vi "Set Monitoring Session.vi"(8 "error in":errorcluster, 9 "Redundant?":bool, 10 "session_rx_monitor":T1[](array[typedef]) {"Strobe" items=["FDX_MON_STROBE_DIS", "FDX_MON_STROBE_STOP", "FDX_MON_STROBE_START"]; "CaptureMode" items=["FDX_MON_SINGLE ", "FDX_MON_CONTINUOUS", "FDX_MON_SELECTIVE", "FDX_MON_RECORDING", "FDX_MON_REROS", "FDX_MON_HMU"]; "DefaultCronoMode" items=["FDX_RX_DEFAULT_ENA_CNT", "FDX_RX_DEFAULT_MON_ENA_ALL", "FDX_RX_DEFAULT_MON_ENA_GOOD"]}, 11 "Port Section Ref in":T2 format="%.0x") -> (0 "error out":errorcluster, 3 "Item Ref out":T2 format="%.0x")   [LabVIEW 2020, in "AIM ARINC 664 Scripting.lvlib"]
uses:
  AIM ARINC 664 Scripting.lvlib
  <vilib>/NI VeriStand/Custom Device API/Custom Device Item Ref.ctl
  <vilib>/NI VeriStand/Custom Device API/Custom Device API.lvlib
  Shared/session_rx_monitor.ctl
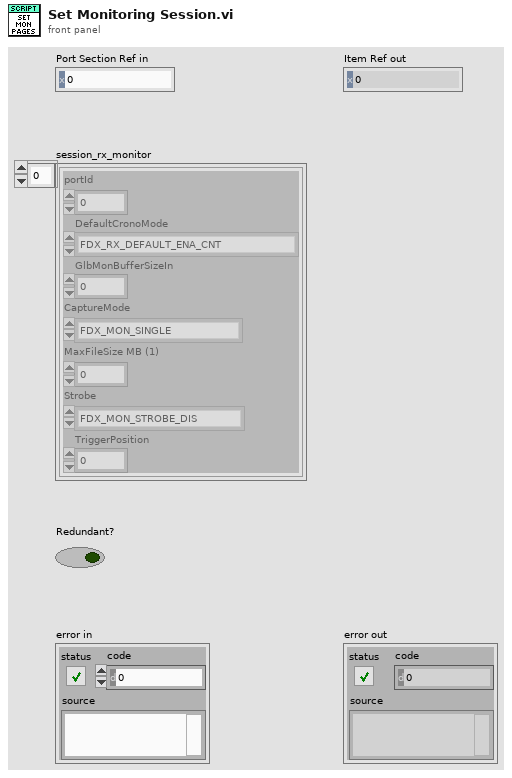
[diagram p1: front panel]
types:
  T1 = typedef "session_rx_monitor.ctl" = cluster{"portId":u32, "DefaultCronoMode":u32, "GlbMonBufferSizeIn":u32, "CaptureMode":u32, "MaxFileSize MB (1)":u32, "Strobe":u32, "TriggerPosition":u32}
  T2 = typedef "Custom Device API.lvlib/Custom Device Item Ref.ctl" = u64
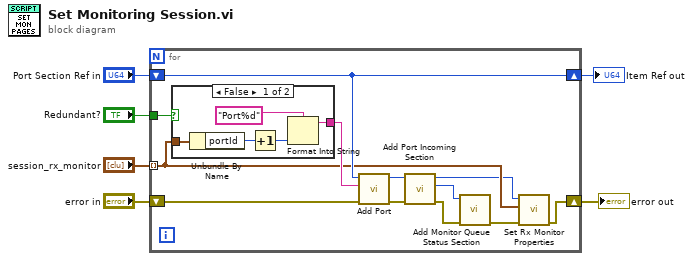
[diagram p0: block diagram]
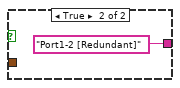
[diagram p2: hidden frame]
diagram:
  n1 = for {
    shift-right: [w9] -> w6
    shift-left: "error in" -> [w13]
    shift-right: [w12] -> w3
    shift-left: "Port Section Ref in" -> [w12]
    tunnel: "session_rx_monitor" -> [w11] mode=indexing
    tunnel: "Redundant?" -> [w7]
    n2 = case shown="False" w7 {
      tunnel: [w23 "Port1-2 [Redundant]"] -> w16
      tunnel: w11 -> [w20 _]
      frame False {
        n3 = Unbundle By Name(w20) -> ("portId"=w21:u32)
        n4 = Increment(x=w21) -> (x+1=w19:u32)
        n5 = Format Into String(format string="Port%d", w19) -> (resulting string=w23:string)  [unwired: 2 in, 1 out]
      }
      frame True {
      }
    }
    n6 = call "Add Port.vi"("error in"=w13, "Port Name"=w16, "Ports Ref"=w12) -> ("error out"=w14:errorcluster, "Port Ref out"=w15:T2)  [unwired: 7 in]
    n7 = call "Add Port Incoming Section.vi"("error in"=w14, "Port Ref"=w15) -> ("error out"=w18:errorcluster, "Section Ptr"=w17:T2, "Port Ref out"=w8:T2)  [unwired: 7 in]
    n8 = call "Add Monitor Queue Status Section.vi"("error in"=w18, "Section ref in"=w17) -> ("error out"=w10:errorcluster)  [unwired: 6 in, 3 out]
    n9 = call "Set Rx Monitor Properties.vi"("error in"=w10, "session_rx_monitor"=w11, "custom device ref in"=w8) -> ("error out"=w9:errorcluster)  [unwired: 7 in, 1 out]
  }
  "error out" <- w6
  "Item Ref out" <- w3
